vi "util_ShutdownTable.vi"(6 "error in":errorcluster, 7 "FPGA VI Reference In":refnum<k20>) -> (1 "Success":bool, 2 "error out":errorcluster, 3 "FPGA VI Reference Out":refnum<k20>)   [LabVIEW 2012]
uses:
  <vilib>/Utility/error.llb/Error Cluster From Error Code.vi
  <vilib>/rvi/errors/niLvFpgaAdjustHostInterfaceError.vi
  <vilib>/rvi/interface/nirviReadWriteControl/nirviReadWriteControl.xnode
  NiFpgaLv.dll
  <vilib>/rvi/interface/Simulation/niFpgaSimulationCallBeginRW.vi
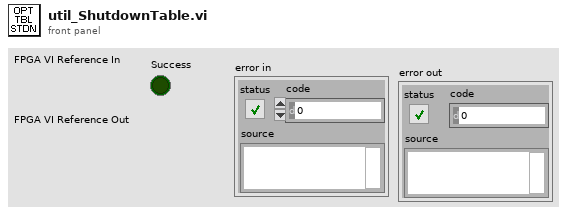
[diagram p1: front panel]
types:
  T1 = cluster{"Pulse Length (Ticks)":u32, "Pulse Period (Ticks)":u32, "Ao (Int)":i32, "Seq 1 (High)":bool, "Seq 2 (Low)":bool}
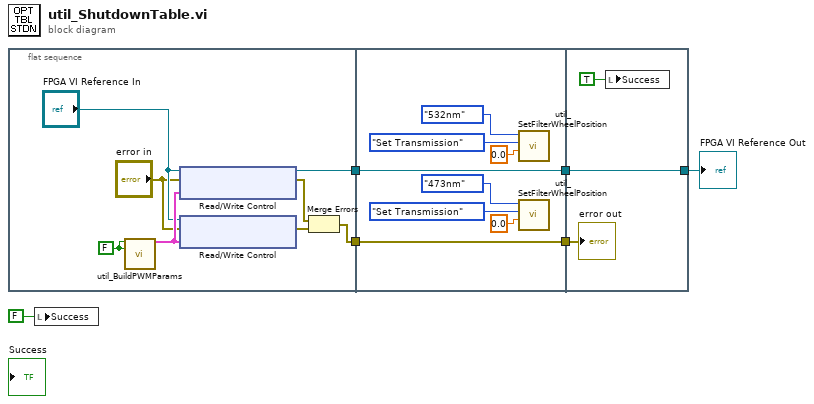
[diagram p0: block diagram]
diagram:
  n1 = flat-sequence {
    tunnel: [w11] -> w4
    tunnel: [w7] -> w1
    tunnel: [w22] -> w5
    tunnel: w4 -> [w22]
    tunnel: [w15] -> w2
    tunnel: w1 -> [w15]
    tunnel: [w24] -> w3
    tunnel: w5 -> [w24]
    tunnel: w2 -> [w23]
    frame #0 {
      w14 = FALSE ("Burst")
      n2 = call "util_BuildPWMParams.vi"("Burst"=w14, "Continous"=w14) -> ("PWM Params"=w13:T1)  [unwired: 13 in]
      n3 = xnode "Read/Write Control"("FPGA VI Reference In"="FPGA VI Reference In", "error in"="error in", "PWM 532nm Laser"=w13) -> ("FPGA VI Reference Out"=w11:refnum<k20>, "error out"=w10:errorcluster)
      n4 = xnode "Read/Write Control"("FPGA VI Reference In"="FPGA VI Reference In", "error in"="error in", "PWM 473nm Laser"=w13) -> ("error out"=w9:errorcluster)  [unwired: 1 out]
      n5 = Merge Errors(w10, w9) -> (w7:errorcluster)
    }
    frame #1 {
      n6 = call "util_SetFilterWheelPosition.vi"("Filter Transmission"=0.0, "Mode"=enum16{"Set Position", "Set Transmission"}."Set Transmission", "Filter Wheel"=enum16{"473nm", "532nm"}."532nm") -> ()  [unwired: 8 in, 1 out]
      n7 = call "util_SetFilterWheelPosition.vi"("Filter Transmission"=0.0, "Mode"=enum16{"Set Position", "Set Transmission"}."Set Transmission", "Filter Wheel"=enum16{"473nm", "532nm"}."473nm") -> ()  [unwired: 8 in, 1 out]
    }
    frame #2 {
      n8 = local write "Success"(TRUE ("Success")) -> ()
      "error out" <- w23
    }
  }
  n9 = local write "Success"(FALSE ("Success")) -> ()
  "FPGA VI Reference Out" <- w3
